vi "Manager Control Panel.vi"() -> ()   [LabVIEW 2024]
uses:
  manager_daemon/manager_daemon.lvclass
  <vilib>/addons/_JKI Toolkits/State Machine/_JKI_lib_State_Machine.llb/Select State(s)_err__jki_lib_state_machine.vi
  <vilib>/addons/_JKI Toolkits/State Machine/_JKI_lib_State_Machine.llb/Periodic Trigger__ogtk__JKI-SM__jki_lib_state_machine.vi
panel:
  in  "save indices":bool
  in  "launch crawler":bool
  in  "launch interface":bool
  in  "launch graphic UI":bool
  in  "generate indices":bool
  in  "Exit":bool
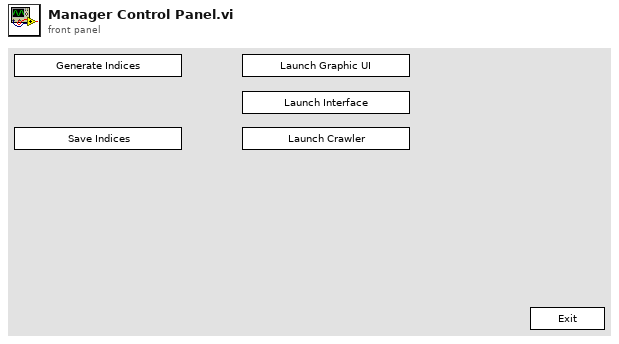
[diagram p1: front panel]
types:
  T1 = enum32{"Invalid", "Standard", "Closed", "Hidden", "Minimized", "Maximized"}
  T2 = enum32{"invalid app kind", "Development System", "Run Time System", "Student Edition", "Embedded LabVIEW", "Evaluation", "Custom"}
  T3 = cluster{"Core":cluster{"Current VI Reference":refnum<vi>, "Close Panel on Exit?":bool}, "manager_daemon":refnum<class "manager_daemon.lvclass">}
  T4 = cluster{"Current VI Reference":refnum<vi>, "Close Panel on Exit?":bool}
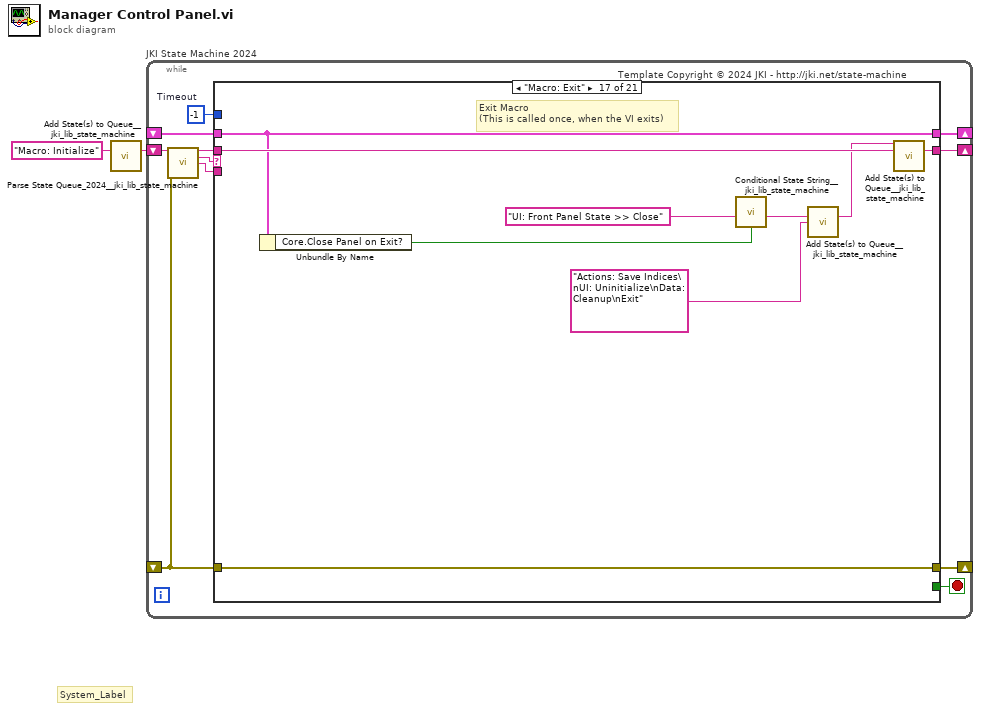
[diagram p0: block diagram]
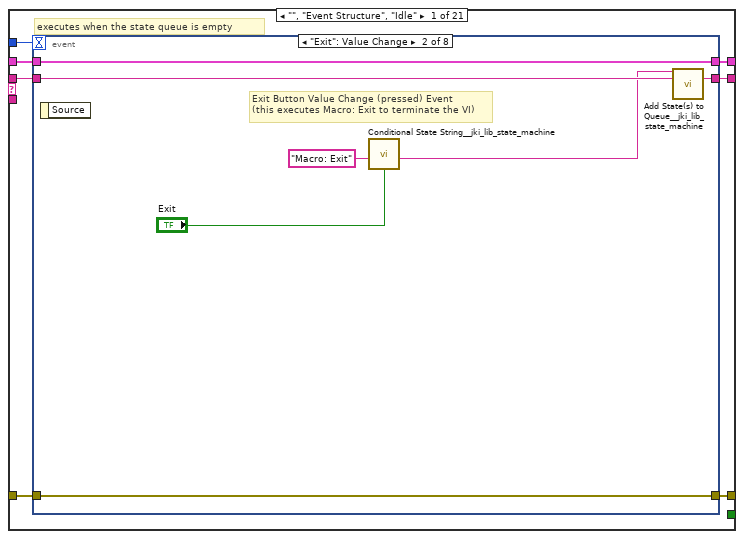
[diagram p2: hidden frame]
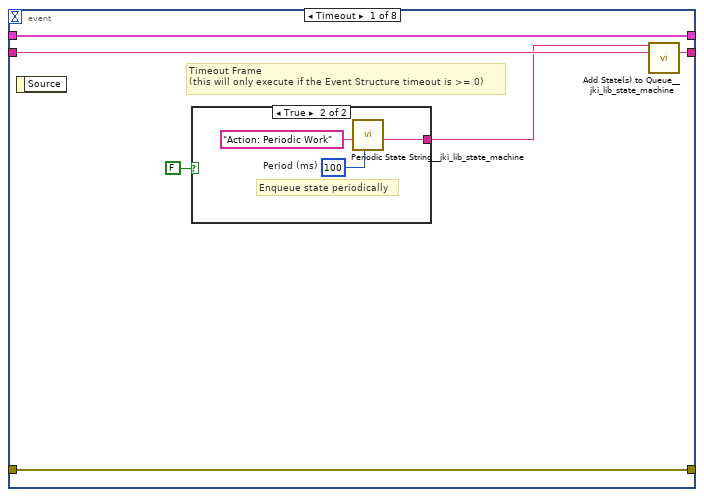
[diagram p3: hidden frame]
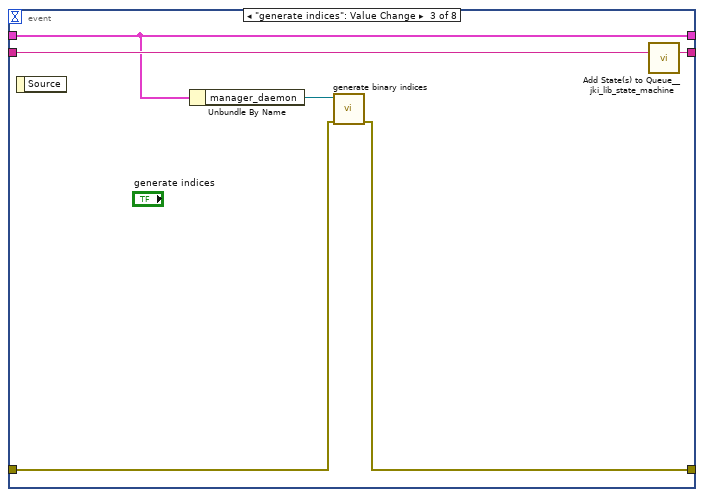
[diagram p5: hidden frame]
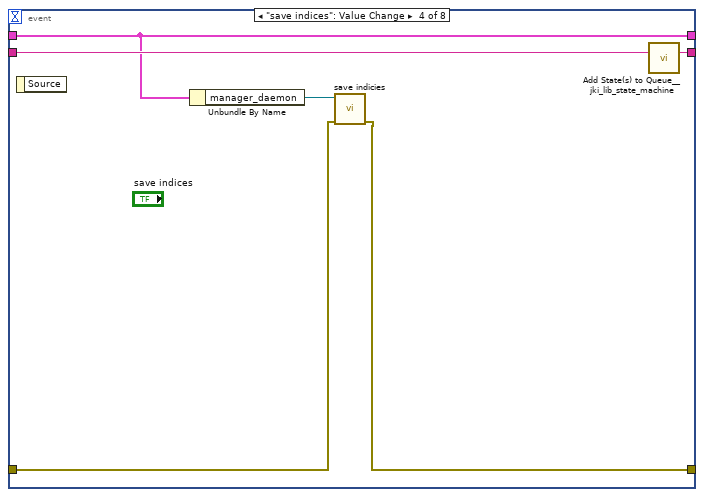
[diagram p6: hidden frame]
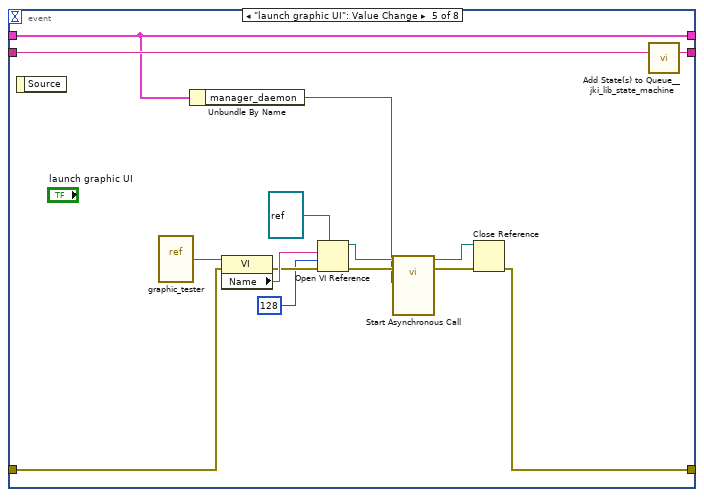
[diagram p7: hidden frame]
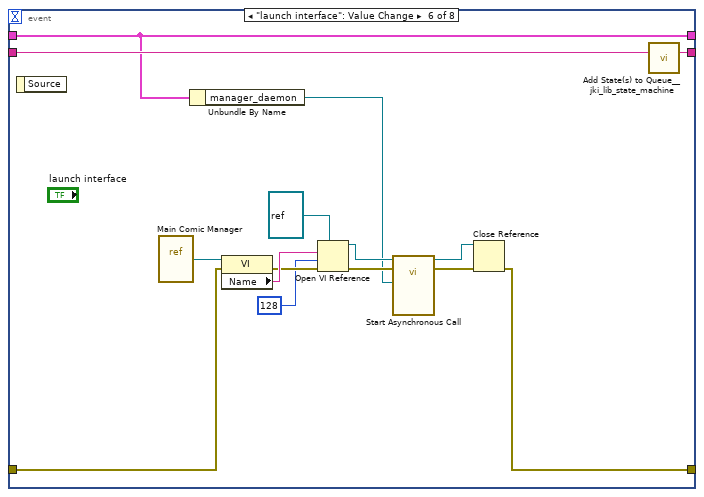
[diagram p8: hidden frame]
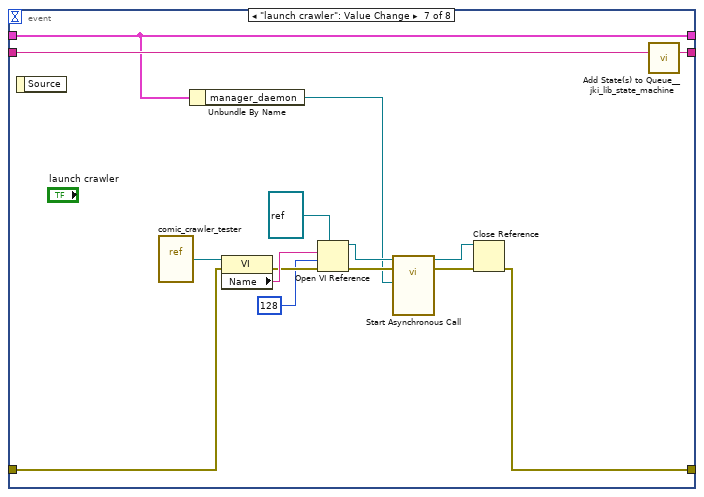
[diagram p9: hidden frame]
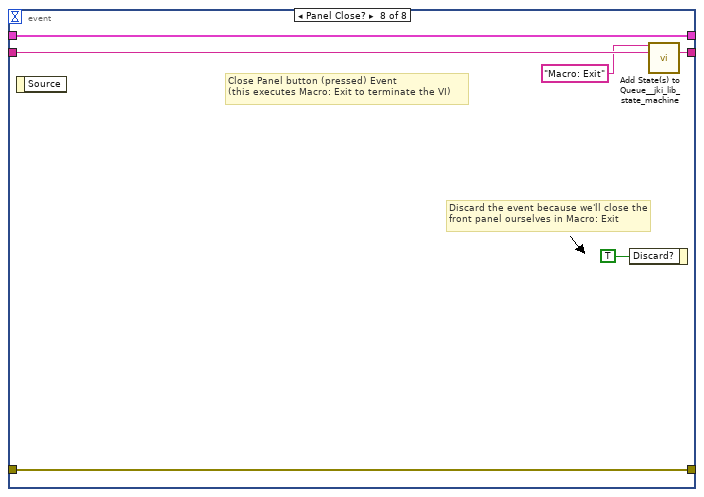
[diagram p10: hidden frame]
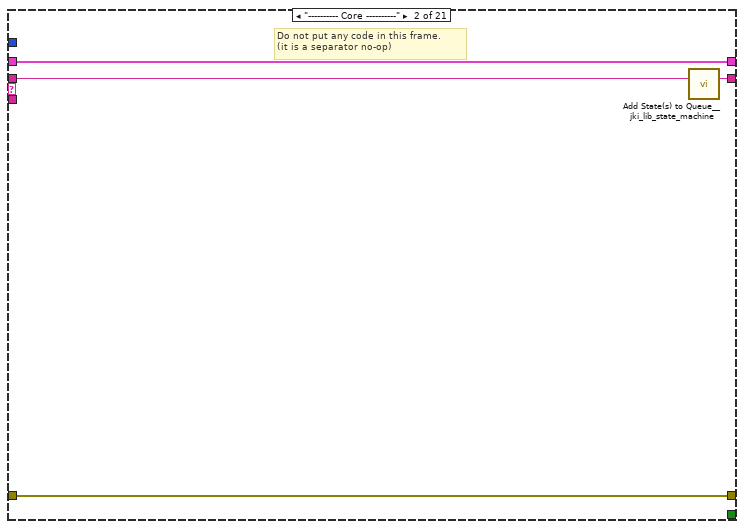
[diagram p11: hidden frame]
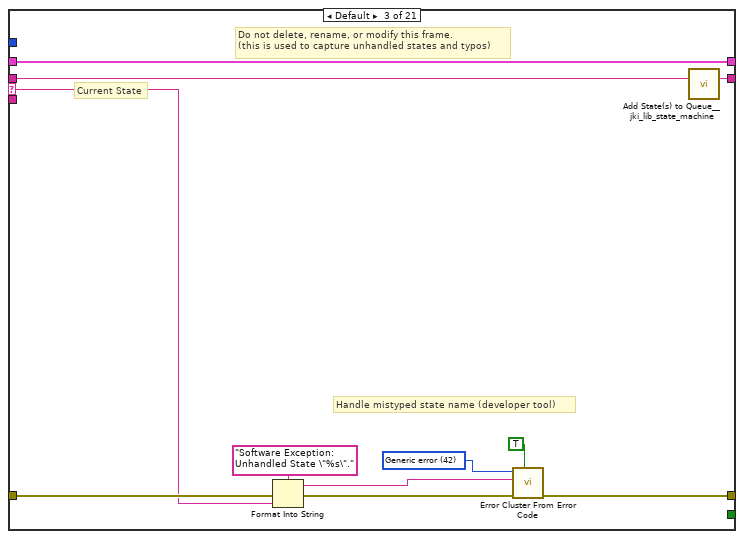
[diagram p12: hidden frame]
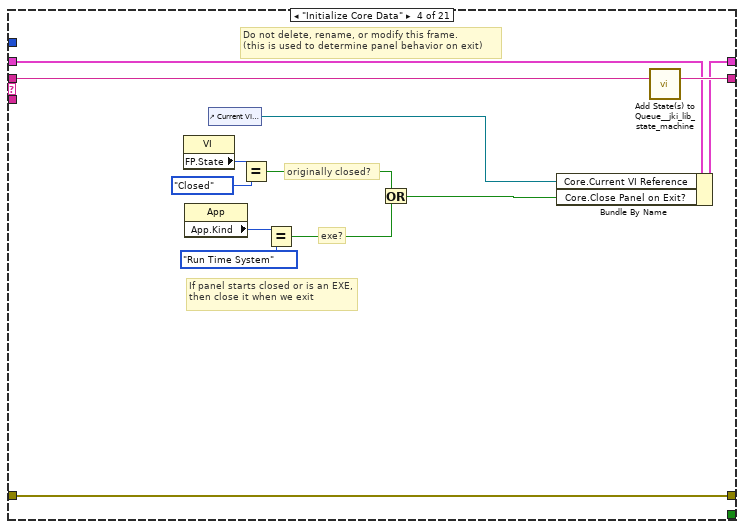
[diagram p13: hidden frame]
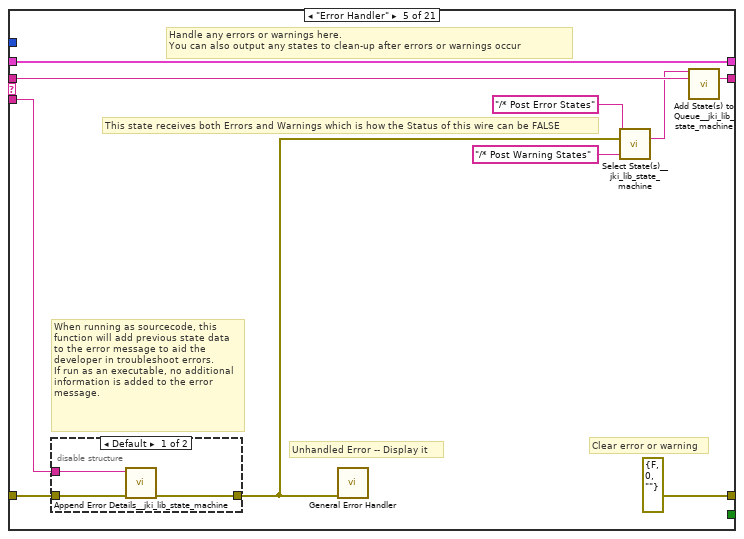
[diagram p14: hidden frame]
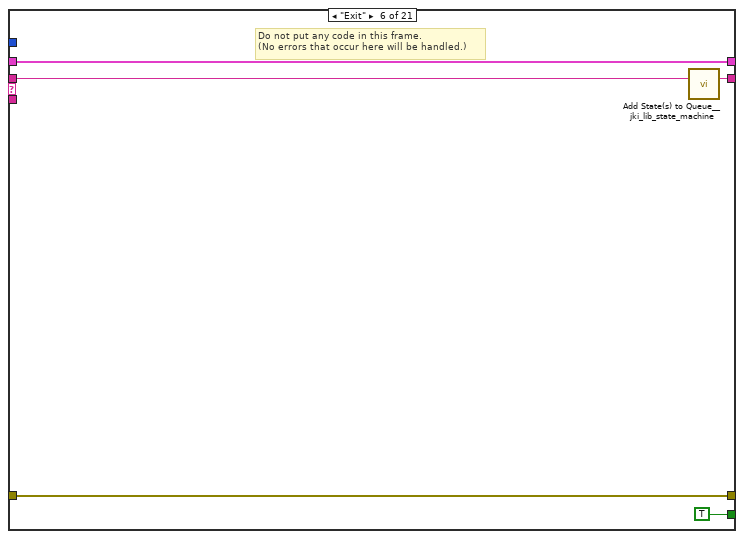
[diagram p16: hidden frame]
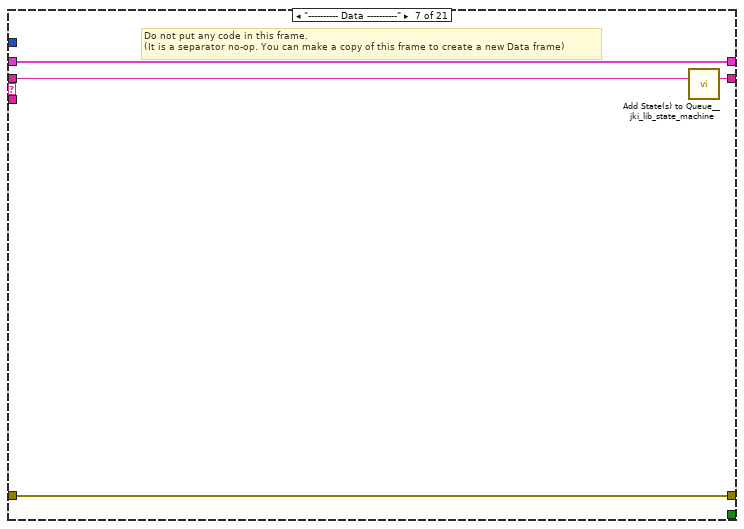
[diagram p17: hidden frame]
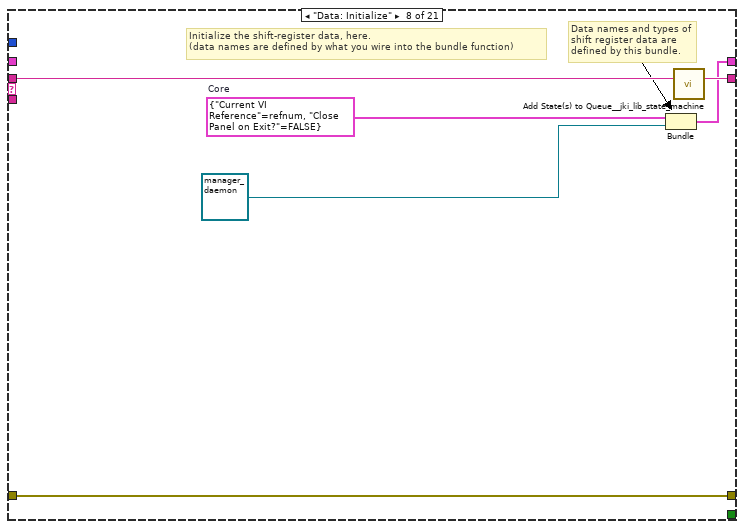
[diagram p18: hidden frame]
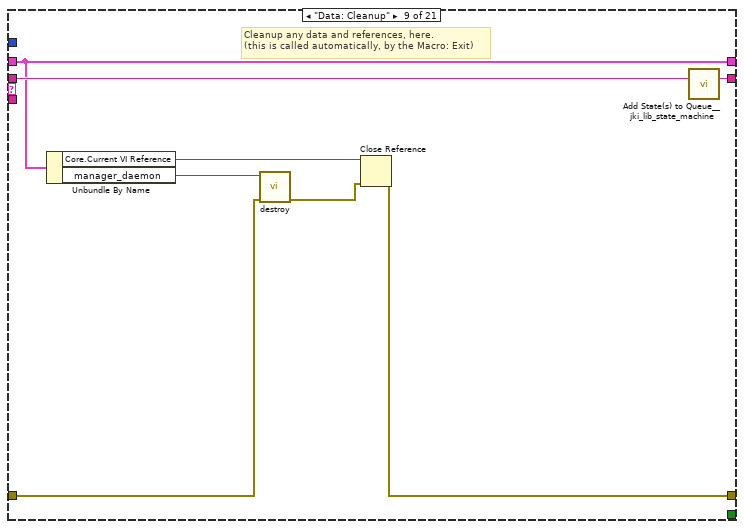
[diagram p19: hidden frame]
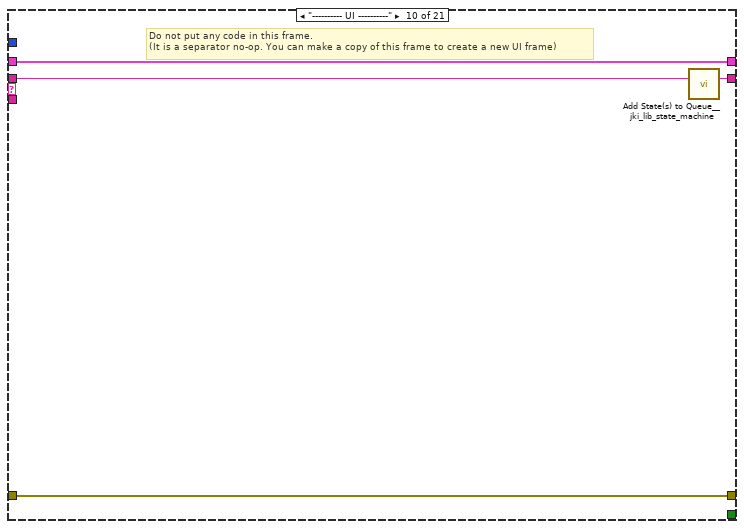
[diagram p20: hidden frame]
diagram:
  # "System_Label"
  n1 = call <vilib>:"Add State(s) to Queue__jki_lib_state_machine.vi"("State(s) in (\"\")"="Macro: Initialize") -> ("States Out"=w2:string)  [unwired: 14 in]
  n2 = while "JKI State Machine 2024" {
    shift-right: [w6] -> _
    shift-left: _ -> [w5]
    shift-right: [w9] -> _
    shift-left: _ -> [w3]
    shift-right: [w8] -> _
    shift-left: w2 -> [w10]
    stop <- w7 stop-if-true
    w4 = -1  # Timeout
    # "Template Copyright © 2024 JKI - http://jki.net/state-machine"
    n3 = call <vilib>:"Parse State Queue_2024__jki_lib_state_machine.vi"("State Queue"=w10, "Error In (no error)"=w3) -> ("Remaining States"=w12:string, "Current State"=w13:string, "Arguments"=w11:string)  [unwired: 11 in]
    n4 = case shown="\"Macro: Exit\"" w13 {
      selector: w13 -> [_ _ w104 _ _ _ _ _ _ _ _ _ _ _ _ _ _ _ _ _ _]
      tunnel: w12 -> [w20 w103 w108 w127 w137 w146 w150 w156 w164 w168 w172 w176 w182 w193 w262 w267 w276 w280 w286 w295 w306]
      tunnel: w11 -> [_ _ _ _ w132 _ _ _ _ _ _ _ w177 w187 _ _ _ _ _ _ _]
      tunnel: w5 -> [w18 w100 w106 w120 w134 w144 w147 _ w160 w165 w170 w174 w180 w189 w259 w264 w274 w277 w284 w292 w298]
      tunnel: [w17 w101 w110 w124 errorcluster {"status"=FALSE, "code"=0, "source"=""} ("error out") w142 w148 w153 w161 w166 w169 w173 w178 w190 w260 w265 w268 w278 w281 w287 w300] -> w9
      tunnel: w3 -> [w14 w101 w109 w124 w133 w142 w148 w153 w157 w166 w169 w173 w179 w191 w260 w265 w268 w278 w282 w293 w299]
      tunnel: [w19 w102 w107 w126 w136 w145 w149 w155 w163 w167 w171 w175 w181 w192 w261 w266 w275 w279 w285 w294 w305] -> w8
      tunnel: [_ _ _ _ _ TRUE _ _ _ _ _ _ _ _ _ _ _ _ _ _ _] -> w7
      tunnel: [w16 w100 w106 w125 w134 w144 w147 w154 w160 w165 w170 w174 w180 w189 w259 w264 w274 w277 w284 w291 w296] -> w6
      tunnel: w4 -> [w15 _ _ _ _ _ _ _ _ _ _ _ _ _ _ _ _ _ _ _ _]
      frame "", "Event Structure", "Idle" {
        # "executes when the state queue is empty"
        n5 = event shown="[1] \"Exit\": Value Change" {
          selector: _ -> [_ _ _ _ _ _ _ _]
          dyn-events: _ -> [_ _ _ _ _ _ _ _]
          timeout: w15 -> [_ _ _ _ _ _ _ _]
          tunnel: w20 -> [w26 w36 w42 w48 w63 w78 w93 w99]
          tunnel: [w25 w35 w41 w47 w62 w77 w92 w98] -> w19
          tunnel: w18 -> [w23 w33 w40 w46 w61 w76 w91 w96]
          tunnel: [w24 w34 w37 w43 w49 w64 w79 w97] -> w17
          tunnel: w14 -> [w24 w34 w38 w44 w51 w66 w81 w97]
          tunnel: [w23 w33 w40 w46 w61 w76 w91 w96] -> w16
          event Timeout {
            # "Timeout Frame\n(this will only execute if the Event Structure timeout is >= 0)"
            n6 = event-data() -> ()  [unwired: 1 in, 1 out]
            n7 = case shown="True" FALSE {
              tunnel: [_ w29] -> w22
              frame False {
              }
              frame True {
                w27 = u32 100  # Period (ms)
                # "Enqueue state periodically"
                n8 = call <vilib>:"Periodic State String__jki_lib_state_machine.vi"("Period (ms)"=w27, "State"="Action: Periodic Work") -> ("State Out"=w29:string)  [unwired: 9 in]
              }
            }
            n9 = call <vilib>:"Add State(s) to Queue__jki_lib_state_machine.vi"("State(s) in Front (\"\")"=w22, "State(s) in (\"\")"=w26) -> ("States Out"=w25:string)  [unwired: 13 in]
          }
          event "Exit": Value Change {
            # "Exit Button Value Change (pressed) Event\n(this executes Macro: Exit to terminate the VI)"
            n10 = event-data() -> ()  [unwired: 1 in, 1 out]
            n11 = call <vilib>:"Conditional State String__jki_lib_state_machine.vi"("Do State(s)?"="Exit", "State"="Macro: Exit") -> ("State Out"=w30:string)  [unwired: 7 in]
            n12 = call <vilib>:"Add State(s) to Queue__jki_lib_state_machine.vi"("State(s) in Front (\"\")"=w30, "State(s) in (\"\")"=w36) -> ("States Out"=w35:string)  [unwired: 13 in]
          }
          event "generate indices": Value Change {
            n13 = event-data() -> ()  [unwired: 1 in, 1 out]
            n14 = Unbundle By Name(w40) -> ("manager_daemon"=w39:refnum<class "manager_daemon.lvclass">)
            n15 = call "generate binary indices.vi"("error in (no error)"=w38, "manager_daemon in"=w39) -> ("error out"=w37:errorcluster)  [unwired: 8 in, 1 out]
            n16 = call <vilib>:"Add State(s) to Queue__jki_lib_state_machine.vi"("State(s) in (\"\")"=w42) -> ("States Out"=w41:string)  [unwired: 14 in]
          }
          event "save indices": Value Change {
            n17 = event-data() -> ()  [unwired: 1 in, 1 out]
            n18 = Unbundle By Name(w46) -> ("manager_daemon"=w45:refnum<class "manager_daemon.lvclass">)
            n19 = call "save indicies.vi"("error in (no error)"=w44, "manager_daemon in"=w45) -> ("error out"=w43:errorcluster)  [unwired: 8 in, 1 out]
            n20 = call <vilib>:"Add State(s) to Queue__jki_lib_state_machine.vi"("State(s) in (\"\")"=w48) -> ("States Out"=w47:string)  [unwired: 14 in]
          }
          event "launch graphic UI": Value Change {
            n21 = event-data() -> ()  [unwired: 1 in, 1 out]
            n22 = vi-ref "graphic_tester.vi"() -> (w53:refnum<vi>)
            n23 = Unbundle By Name(w61) -> ("manager_daemon"=w50:refnum<class "manager_daemon.lvclass">)
            n24 = property class="VI"(reference=w53, error in=w51) -> (error out=w54:errorcluster, "Name"=w55:string)  [unwired: 1 out]
            n25 = Open VI Reference(type specifier VI Refnum (for type only)=refnum<vi> refnum, vi path=w55, options=128, error in (no error)=w54) -> (vi reference=w57:refnum<vi>, error out=w60:errorcluster)  [unwired: 2 in]
            n26 = call-by-ref "Start Asynchronous Call"(reference=w57, error in=w60, "manager_daemon"=w50) -> (reference out=w58:refnum<vi>, error out=w59:errorcluster)  [unwired: 11 in]
            n27 = Close Reference(reference=w58, error in (no error)=w59) -> (error out=w49:errorcluster)
            n28 = call <vilib>:"Add State(s) to Queue__jki_lib_state_machine.vi"("State(s) in (\"\")"=w63) -> ("States Out"=w62:string)  [unwired: 14 in]
          }
          event "launch interface": Value Change {
            n29 = event-data() -> ()  [unwired: 1 in, 1 out]
            n30 = vi-ref "Main Comic Manager.vi"() -> (w68:refnum<vi>)
            n31 = Unbundle By Name(w76) -> ("manager_daemon"=w65:refnum<class "manager_daemon.lvclass">)
            n32 = property class="VI"(reference=w68, error in=w66) -> (error out=w69:errorcluster, "Name"=w70:string)  [unwired: 1 out]
            n33 = Open VI Reference(type specifier VI Refnum (for type only)=refnum<vi> refnum, vi path=w70, options=128, error in (no error)=w69) -> (vi reference=w72:refnum<vi>, error out=w75:errorcluster)  [unwired: 2 in]
            n34 = call-by-ref "Start Asynchronous Call"(reference=w72, error in=w75, "manager_daemon"=w65) -> (reference out=w73:refnum<vi>, error out=w74:errorcluster)  [unwired: 11 in]
            n35 = Close Reference(reference=w73, error in (no error)=w74) -> (error out=w64:errorcluster)
            n36 = call <vilib>:"Add State(s) to Queue__jki_lib_state_machine.vi"("State(s) in (\"\")"=w78) -> ("States Out"=w77:string)  [unwired: 14 in]
          }
          event "launch crawler": Value Change {
            n37 = event-data() -> ()  [unwired: 1 in, 1 out]
            n38 = vi-ref "comic_crawler_tester.vi"() -> (w83:refnum<vi>)
            n39 = Unbundle By Name(w91) -> ("manager_daemon"=w80:refnum<class "manager_daemon.lvclass">)
            n40 = property class="VI"(reference=w83, error in=w81) -> (error out=w84:errorcluster, "Name"=w85:string)  [unwired: 1 out]
            n41 = Open VI Reference(type specifier VI Refnum (for type only)=refnum<vi> refnum, vi path=w85, options=128, error in (no error)=w84) -> (vi reference=w87:refnum<vi>, error out=w90:errorcluster)  [unwired: 2 in]
            n42 = call-by-ref "Start Asynchronous Call"(reference=w87, error in=w90, "manager_daemon"=w80) -> (reference out=w88:refnum<vi>, error out=w89:errorcluster)  [unwired: 11 in]
            n43 = Close Reference(reference=w88, error in (no error)=w89) -> (error out=w79:errorcluster)
            n44 = call <vilib>:"Add State(s) to Queue__jki_lib_state_machine.vi"("State(s) in (\"\")"=w93) -> ("States Out"=w92:string)  [unwired: 14 in]
          }
          event Panel Close? {
            # "Discard the event because we'll close the front panel ourselves in Macro: Exit"
            # "Close Panel button (pressed) Event\n(this executes Macro: Exit to terminate the VI)"
            n45 = event-data() -> ()  [unwired: 1 in, 1 out]
            n46 = event-data("Discard?"=TRUE) -> ()  [unwired: 1 in, 1 out]
            n47 = call <vilib>:"Add State(s) to Queue__jki_lib_state_machine.vi"("State(s) in Front (\"\")"="Macro: Exit", "State(s) in (\"\")"=w99) -> ("States Out"=w98:string)  [unwired: 13 in]
          }
        }
      }
      frame "---------- Core ----------" {
        # "Do not put any code in this frame.\n(it is a separator no-op)"
        n48 = call <vilib>:"Add State(s) to Queue__jki_lib_state_machine.vi"("State(s) in (\"\")"=w103) -> ("States Out"=w102:string)  [unwired: 14 in]
      }
      frame Default {
        w113 = 42 items=["No error", "Argument error", "Memory is full", "Out of zone", "End of file", "File already open", "Generic file I/O error", "File not found", "File permission error", "Disk is full", "Duplicate path", "Too many files open", "System feature not enabled", "Resource file not found", "Cannot add resource", "Resource not found", "Image not found", "Image memory error", "Pen does not exist", "Config type invalid", "Config token not found", "Config parse error", "Config memory error", "Bad external code format", "Bad external code offset", "External code not present", "Null window", "Destroy window error", "Null menu", "Print aborted", "Bad print record", "Print driver error", "Windows error during printing", "Memory error during printing", "Print dialog error", "Generic print error", "Invalid device refnum", "Device not found", "Device parameter error", "Device unit error", "Cannot open device", "Device call aborted", "Generic error", "Cancelled by user", "Object ID too low", "Object ID too high", "Object not in heap", "Unknown heap", "Unknown object (invalid DefProc)", "Unknown object (DefProc not in table)", "Message out of range", "Invalid (null) method", "Unknown message", "Manager call not supported", "Bad address", "Network operation in progress", "Network operation timed out", "Connection is busy", "Network attribute not supported", "Network error", "Address in use", "System out of memory", "Connection aborted", "Connection refused", "Not connected", "Already connected", "Connection closed", "Initialization error (interapplication manager)", "Bad occurrence", "Wait on unbound occurrence handler", "Occurrence queue overflow", "Datalog type conflict", "Unused", "Unrecognized type (interapplication manager)", "Memory corrupt", "Failed to make temporary DLL", "Old CIN version", "Drag socket not found", "Failed to load drop-object", "Failed to register OLE object", "Failed to release OLE object", "Format specifier type mismatch", "Unknown format specifier", "Too few format specifiers", "Too many format specifiers", "Scan failed", "Newer CIN version", "Error converting to variant", "Runtime menu error", "Password tampered", "Variant attribute not found", "Incompatible variant data type", "Event data is not available", "Event Store is not present", "Occurrence is not found", "Event Queue is not created", "Event info is not available", "Refnum passed is NULL", "Error retrieving Class GUID", "Error retrieving CoClass GUID", "Error retrieving TypeLib GUID.", "Bad built application magic bytes.", "Specific driver is different from the specific driver associated with the Logical Name.", "There is no session opened to the class driver.", "Max Error", "MAX - Error with config objects", "MAX - Error loading configuration", "MAX - Group not supported"]
        # "Current State"
        # "Do not delete, rename, or modify this frame.\n(this is used to capture unhandled states and typos)"
        # "Handle mistyped state name (developer tool)"
        n49 = Format Into String(format string="Software Exception: Unhandled State \"%s\"." ("message"), error in=w109, w104) -> (resulting string=w112:string, error out=w111:errorcluster)  [unwired: 1 in]
        n50 = call <vilib>:"Error Cluster From Error Code.vi"("show call chain? (False)"=TRUE, "error in (no error)"=w111, "error message (\"\")"=w112, "error code (0)"=w113) -> ("error out"=w110:errorcluster)  [unwired: 5 in]
        n51 = call <vilib>:"Add State(s) to Queue__jki_lib_state_machine.vi"("State(s) in (\"\")"=w108) -> ("States Out"=w107:string)  [unwired: 14 in]
      }
      frame "Initialize Core Data" {
        # "Do not delete, rename, or modify this frame.\n(this is used to determine panel behavior on exit)"
        # "originally closed?"
        # "exe?"
        # "If panel starts closed or is an EXE, then close it when we exit"
        n52 = property class="VI"() -> ("FP.State"=w117:T1)  [unwired: 2 in, 2 out]
        n53 = property class="App"() -> ("App.Kind"=w123:T2)  [unwired: 2 in, 2 out]
        n54 = control-ref of="Current VI Reference"() -> (w118:refnum<vi>)
        n55 = Equal?(x=w117, y=T1."Closed" ("Front Panel Window:State")) -> (x = y?=w115:bool)
        n56 = Equal?(x=w123, y=T2."Run Time System" ("Application:Kind")) -> (x = y?=w121:bool)
        n57 = Or(x=w115, y=w121) -> (x .or. y?=w119:bool)
        n58 = Bundle By Name(cluster=w120, "Core.Current VI Reference"=w118, "Core.Close Panel on Exit?"=w119) -> (w125:T3)
        n59 = call <vilib>:"Add State(s) to Queue__jki_lib_state_machine.vi"("State(s) in (\"\")"=w127) -> ("States Out"=w126:string)  [unwired: 14 in]
      }
      frame "Error Handler" {
        # "When running as sourcecode, this function will add previous state data to the error message to aid the developer in troubleshoot errors.\nIf run as an executable, no additional information is added to the error message."
        # "This state receives both Errors and Warnings which is how the Status of this wire can be FALSE"
        # "Unhandled Error -- Display it"
        # "Handle any errors or warnings here.\nYou can also output any states to clean-up after errors or warnings occur"
        # "Clear error or warning"
        n60 = disable-structure shown="Default" {
          disable-tunnel: w133 -> [w140 w141]
          disable-tunnel: w132 -> [w139 _]
          disable-tunnel: [w138 w141] -> w131
          frame condition #0 (active) {
            n61 = call <vilib>:"Append Error Details__jki_lib_state_machine.vi"("error in (no error)"=w140, "Previous State and Argument(s)"=w139) -> ("error out"=w138:errorcluster)  [unwired: 9 in]
          }
          frame condition #1 {
          }
        }
        n62 = call <vilib>:"General Error Handler.vi"("error in (no error)"=w131) -> ()  [unwired: 10 in, 5 out]
        n63 = call-poly <vilib>:"Select State(s)__jki_lib_state_machine.vi"("State(s) if True (\"\")"="/* Post Error States", "Select"=w131, "State(s) if False (\"\")"="/* Post Warning States") -> ("States Out"=w129:string)  [unwired: 12 in]
        n64 = call <vilib>:"Add State(s) to Queue__jki_lib_state_machine.vi"("State(s) in Front (\"\")"=w129, "State(s) in (\"\")"=w137) -> ("States Out"=w136:string)  [unwired: 13 in]
      }
      frame "Exit" {
        # "Do not put any code in this frame.\n(No errors that occur here will be handled.)"
        n65 = call <vilib>:"Add State(s) to Queue__jki_lib_state_machine.vi"("State(s) in (\"\")"=w146) -> ("States Out"=w145:string)  [unwired: 14 in]
      }
      frame "---------- Data ----------" {
        # "Do not put any code in this frame.\n(It is a separator no-op. You can make a copy of this frame to create a new Data frame)"
        n66 = call <vilib>:"Add State(s) to Queue__jki_lib_state_machine.vi"("State(s) in (\"\")"=w150) -> ("States Out"=w149:string)  [unwired: 14 in]
      }
      frame "Data: Initialize" {
        w152 = T4 {"Current VI Reference"=refnum, "Close Panel on Exit?"=FALSE}  # Core
        # "Data names and types of shift register data are defined by this bundle."
        # "Initialize the shift-register data, here.\n(data names are defined by what you wire into the bundle function)"
        n67 = Bundle("Core"=w152, "manager_daemon"=refnum<class "manager_daemon.lvclass"> refnum) -> (w154:T3)  [unwired: 1 in]
        n68 = call <vilib>:"Add State(s) to Queue__jki_lib_state_machine.vi"("State(s) in (\"\")"=w156) -> ("States Out"=w155:string)  [unwired: 14 in]
      }
      frame "Data: Cleanup" {
        # "Cleanup any data and references, here.\n(this is called automatically, by the Macro: Exit)"
        n69 = Unbundle By Name(w160) -> ("Core.Current VI Reference"=w162:refnum<vi>, "manager_daemon"=w159:refnum<class "manager_daemon.lvclass">)
        n70 = call "destroy.vi"("error in (no error)"=w157, "manager_daemon in"=w159) -> ("error out"=w158:errorcluster)  [unwired: 8 in, 1 out]
        n71 = Close Reference(reference=w162, error in (no error)=w158) -> (error out=w161:errorcluster)
        n72 = call <vilib>:"Add State(s) to Queue__jki_lib_state_machine.vi"("State(s) in (\"\")"=w164) -> ("States Out"=w163:string)  [unwired: 14 in]
      }
      frame "---------- UI ----------" {
        # "Do not put any code in this frame.\n(It is a separator no-op. You can make a copy of this frame to create a new UI frame)"
        n73 = call <vilib>:"Add State(s) to Queue__jki_lib_state_machine.vi"("State(s) in (\"\")"=w168) -> ("States Out"=w167:string)  [unwired: 14 in]
      }
      frame "UI: Initialize" {
        # "Initialize the User Interface, here.\n(this is called automatically, by the Macro: Initialize)"
        n74 = call <vilib>:"Add State(s) to Queue__jki_lib_state_machine.vi"("State(s) in (\"\")"=w172) -> ("States Out"=w171:string)  [unwired: 14 in]
      }
      frame "UI: Uninitialize" {
        # "Cleanup the User Interface, here.\n(this is called automatically, by the Macro: Exit)"
        n75 = call <vilib>:"Add State(s) to Queue__jki_lib_state_machine.vi"("State(s) in (\"\")"=w176) -> ("States Out"=w175:string)  [unwired: 14 in]
      }
      frame "UI: Cursor Set" {
        # "Argument"
        # "Set and Unset Cursor Busy.\n(Usage: \"UI: Cursor Set >> Busy|Idle\")"
        n76 = case shown="\"Idle\", Default" w177 {
          tunnel: w179 -> [w184 w186]
          tunnel: [w183 w185] -> w178
          frame "Idle", Default {
            n77 = call <vilib>:"Unset Busy.vi"("error in (no error)"=w184) -> ("error out"=w183:errorcluster)  [unwired: 10 in]
          }
          frame "Busy" {
            n78 = call <vilib>:"Set Busy.vi"("error in (no error)"=w186) -> ("error out"=w185:errorcluster)  [unwired: 9 in, 1 out]
          }
        }
        n79 = call <vilib>:"Add State(s) to Queue__jki_lib_state_machine.vi"("State(s) in (\"\")"=w182) -> ("States Out"=w181:string)  [unwired: 14 in]
      }
      frame "UI: Front Panel State" {
        # "Argument"
        # "Set Front Panel Open or Closed\n(Usage: \"UI: Front Panel State >> Open|Close\")"
        n80 = Unbundle By Name(w189) -> ("Core.Current VI Reference"=w188:refnum<vi>)
        n81 = case shown="\"Minimize\", \"Minimized\"" w187 {
          tunnel: w191 -> [w199 w214 w225 w238 w251]
          tunnel: [w201 w215 w227 w240 w253] -> w190
          tunnel: w188 -> [w200 w212 w226 w239 w252]
          frame "Open", "Standard", Default {
            w194 = T1."Standard" ("State")
            n82 = property class="VI"(reference=w200, error in=w199) -> (reference out=w197:refnum<vi>, error out=w198:errorcluster, "FP.State"=w196:T1)
            n83 = Not Equal?(x=w196, y=w194) -> (x != y?=w195:bool)
            n84 = case shown="True" w195 {
              tunnel: [w205 w207] -> w201
              tunnel: w198 -> [w204 w207]
              tunnel: w197 -> [w203 _]
              tunnel: w194 -> [w202 _]
              frame True {
                n85 = invoke class="VI" method="FP.Open"(reference=w203, error in=w204, "Activate"=TRUE, "State"=w202) -> (error out=w205:errorcluster)  [unwired: 1 in, 4 out]
              }
              frame False {
              }
            }
          }
          frame "Close", "Closed" {
            n86 = property class="VI"(reference=w212, error in=w214) -> (reference out=w211:refnum<vi>, error out=w213:errorcluster, "FP.State"=w209:T1)
            n87 = Not Equal?(x=w209, y=T1."Closed" ("Front Panel Window:State")) -> (x != y?=w208:bool)
            n88 = case shown="True" w208 {
              tunnel: [w216 w219] -> w215
              tunnel: w213 -> [w216 w218]
              tunnel: w211 -> [_ w217]
              frame False {
              }
              frame True {
                n89 = invoke class="VI" method="FP.Close"(reference=w217, error in=w218) -> (error out=w219:errorcluster)  [unwired: 1 in, 2 out]
              }
            }
          }
          frame "Hidden", "Hide" {
            w220 = T1."Hidden" ("State")
            n90 = property class="VI"(reference=w226, error in=w225) -> (reference out=w223:refnum<vi>, error out=w224:errorcluster, "FP.State"=w222:T1)
            n91 = Not Equal?(x=w222, y=w220) -> (x != y?=w221:bool)
            n92 = case shown="True" w221 {
              tunnel: [w231 w232] -> w227
              tunnel: w224 -> [w230 w232]
              tunnel: w223 -> [w229 _]
              tunnel: w220 -> [w228 _]
              frame True {
                n93 = invoke class="VI" method="FP.Open"(reference=w229, error in=w230, "State"=w228) -> (error out=w231:errorcluster)  [unwired: 2 in, 4 out]
              }
              frame False {
              }
            }
          }
          frame "Minimize", "Minimized" {
            w233 = T1."Minimized" ("State")
            n94 = property class="VI"(reference=w239, error in=w238) -> (reference out=w236:refnum<vi>, error out=w237:errorcluster, "FP.State"=w235:T1)
            n95 = Not Equal?(x=w235, y=w233) -> (x != y?=w234:bool)
            n96 = case shown="True" w234 {
              tunnel: [w244 w245] -> w240
              tunnel: w237 -> [w243 w245]
              tunnel: w236 -> [w242 _]
              tunnel: w233 -> [w241 _]
              frame True {
                n97 = invoke class="VI" method="FP.Open"(reference=w242, error in=w243, "State"=w241) -> (error out=w244:errorcluster)  [unwired: 2 in, 4 out]
              }
              frame False {
              }
            }
          }
          frame "Maximize", "Maximized" {
            w246 = T1."Maximized" ("State")
            n98 = property class="VI"(reference=w252, error in=w251) -> (reference out=w249:refnum<vi>, error out=w250:errorcluster, "FP.State"=w248:T1)
            n99 = Not Equal?(x=w248, y=w246) -> (x != y?=w247:bool)
            n100 = case shown="True" w247 {
              tunnel: [w257 w258] -> w253
              tunnel: w250 -> [w256 w258]
              tunnel: w249 -> [w255 _]
              tunnel: w246 -> [w254 _]
              frame True {
                n101 = invoke class="VI" method="FP.Open"(reference=w255, error in=w256, "State"=w254) -> (error out=w257:errorcluster)  [unwired: 2 in, 4 out]
              }
              frame False {
              }
            }
          }
        }
        n102 = call <vilib>:"Add State(s) to Queue__jki_lib_state_machine.vi"("State(s) in (\"\")"=w193) -> ("States Out"=w192:string)  [unwired: 14 in]
      }
      frame "---------- Macro ----------" {
        # "Do not put any code in this frame.\n(It is a separator no-op. You can make a copy of this frame to create a new Macro frame)"
        n103 = call <vilib>:"Add State(s) to Queue__jki_lib_state_machine.vi"("State(s) in (\"\")"=w262) -> ("States Out"=w261:string)  [unwired: 14 in]
      }
      frame "Macro: Initialize" {
        w263 = "Data: Initialize\nInitialize Core Data\nUI: Initialize\nUI: Front Panel State >> Open\nActions: Start Manager"  # Data: Initialize Initialize Core Data UI: Initialize UI: Front Panel State >> Open Actions: Start Manager
        # "Initialization Macro\n(This is called once, when the VI starts)"
        n104 = call <vilib>:"Add State(s) to Queue__jki_lib_state_machine.vi"("State(s) in Front (\"\")"=w263, "State(s) in (\"\")"=w267) -> ("States Out"=w266:string)  [unwired: 13 in]
      }
      frame "Macro: Exit" {
        # "Exit Macro\n(This is called once, when the VI exits)"
        n105 = Unbundle By Name(w274) -> ("Core.Close Panel on Exit?"=w270:bool)
        n106 = call <vilib>:"Conditional State String__jki_lib_state_machine.vi"("Do State(s)?"=w270, "State"="UI: Front Panel State >> Close") -> ("State Out"=w269:string)  [unwired: 7 in]
        n107 = call <vilib>:"Add State(s) to Queue__jki_lib_state_machine.vi"("State(s) in (\"\")"=w269, "State(s) at Back (\"\")"="Actions: Save Indices\nUI: Uninitialize\nData: Cleanup\nExit") -> ("States Out"=w272:string)  [unwired: 13 in]
        n108 = call <vilib>:"Add State(s) to Queue__jki_lib_state_machine.vi"("State(s) in Front (\"\")"=w272, "State(s) in (\"\")"=w276) -> ("States Out"=w275:string)  [unwired: 13 in]
      }
      frame "---------- Actions ----------" {
        # "Template Separator\n(You can make a copy of, or modify, this frame)"
        n109 = call <vilib>:"Add State(s) to Queue__jki_lib_state_machine.vi"("State(s) in (\"\")"=w280) -> ("States Out"=w279:string)  [unwired: 14 in]
      }
      frame "Actions: Save Indices" {
        n110 = Unbundle By Name(w284) -> ("manager_daemon"=w283:refnum<class "manager_daemon.lvclass">)
        n111 = call "save indicies.vi"("error in (no error)"=w282, "manager_daemon in"=w283) -> ("error out"=w281:errorcluster)  [unwired: 8 in, 1 out]
        n112 = call <vilib>:"Add State(s) to Queue__jki_lib_state_machine.vi"("State(s) in (\"\")"=w286) -> ("States Out"=w285:string)  [unwired: 14 in]
      }
      frame "Actions: Start Manager Daemon" {
        n113 = call "create.vi"("error in (no error)"=w293) -> ("error out"=w290:errorcluster, "manager_daemon out"=w289:refnum<class "manager_daemon.lvclass">)  [unwired: 9 in]
        n114 = call "start.vi"("error in (no error)"=w290, "manager_daemon in"=w289) -> ("error out"=w287:errorcluster, "manager_daemon out"=w288:refnum<class "manager_daemon.lvclass">)  [unwired: 8 in]
        n115 = Bundle By Name(cluster=w292, "manager_daemon"=w288) -> (w291:T3)
        n116 = call <vilib>:"Add State(s) to Queue__jki_lib_state_machine.vi"("State(s) in (\"\")"=w295) -> ("States Out"=w294:string)  [unwired: 14 in]
      }
      frame "Actions: Start Manager" {
        n117 = call "create.vi"("error in (no error)"=w299) -> ("error out"=w302:errorcluster, "manager_daemon out"=w304:refnum<class "manager_daemon.lvclass">)  [unwired: 9 in]
        n118 = call "start.vi"("error in (no error)"=w302, "manager_daemon in"=w304) -> ("error out"=w301:errorcluster, "manager_daemon out"=w303:refnum<class "manager_daemon.lvclass">)  [unwired: 8 in]
        n119 = call "load indices.vi"("error in (no error)"=w301, "manager_daemon in"=w303) -> ("error out"=w300:errorcluster, "manager_daemon out"=w297:refnum<class "manager_daemon.lvclass">)  [unwired: 8 in]
        n120 = Bundle By Name(cluster=w298, "manager_daemon"=w297) -> (w296:T3)
        n121 = call <vilib>:"Add State(s) to Queue__jki_lib_state_machine.vi"("State(s) in (\"\")"=w306) -> ("States Out"=w305:string)  [unwired: 14 in]
      }
    }
  }
